vi "PE Get Wavelength.vi"(8 "error in (no error)":errorcluster, 11 "peHandle":u32) -> (0 "error out":errorcluster, 3 "wavelength":dbl)   [LabVIEW 2017, in "PE_Filter_SDK.lvlib"]
doc: "PEFILTERSDK_API PE_STATUS PE_GetWavelength(CPE_HANDLE peHandle, double* wavelength);"
uses:
  PE_Filter_SDK.lvlib
  PE_Filter_SDK.dll
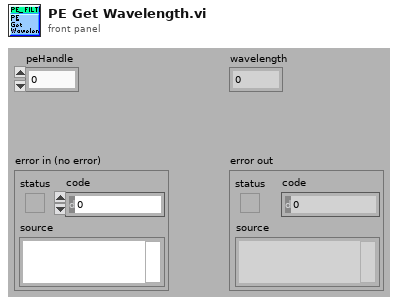
[diagram p1: front panel]
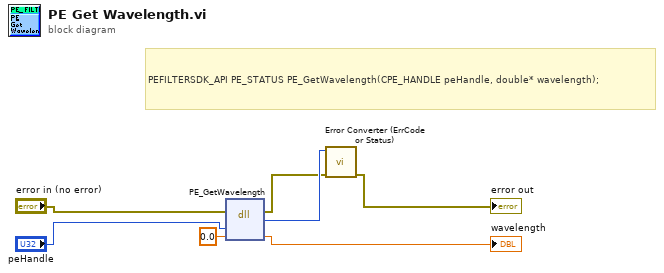
[diagram p0: block diagram]
diagram:
  # "PEFILTERSDK_API PE_STATUS PE_GetWavelength(CPE_HANDLE peHandle, double* wavelength);"
  n1 = dll-call lib="PE_Filter_SDK.*" fn="PE_GetWavelength"(error in="error in (no error)", "peHandle"="peHandle", "wavelength"=0.0) -> (error out=w2:errorcluster, w3:u32, "wavelength"=→"wavelength":dbl)  [unwired: 3 in, 1 out]
  n2 = call "Error Converter (ErrCode or Status).vi"("error in (no error)"=w2, "error code"=w3) -> ("error out"=→"error out":errorcluster)  [unwired: 9 in]
